vi "Main.vi"(10 "DAQ Type":enum16{"Hardware", "Simulation"}(ring), 11 "Module Admin":refnum<class "Delacor_lib_QMH_Module Admin.lvclass">) -> ()   [LabVIEW 2021, in "Serial Hardware.lvlib"]
doc: "This template is based off of the Queued Message Handler design pattern and the Queued Message Handler project template that ships with LabVIEW.\n\nThe main difference is that the queue is private to this module and communication between modules is performed via Broadcast and Request events.\n\nRequest events are wrapped in public API methods and are handled in the Event Handling Loop (EHL) of this VI. Any module can register for Broadcast events sent by this module. The EHL generates messages based on user interface actions.\n\nThe Message Handling Loop (MHL) processes messages generated by the EHL, or by other messages. The messages are string values, so new messages can be added easily to the Message Cases case structure in the MHL. Each message cluster can also provide an optional value for Message Data, which is a variant that can be converted to whatever message-specific data is required.\n_____\nBased on DQMH Project Template 6.1.0.94."
uses:
  Serial Hardware.lvlib
  <vilib>/Delacor/Delacor QMH/Libraries/Module Admin_class/Delacor_lib_QMH_Module Admin.lvclass
  Class/Serial Device/Serial Device.lvclass
  C:/repository/common_ATE/Libraries/Serial Hardware/Class/Abstract/Abstract.lvclass
  Message Data.ctl
  Class/Abstract/Abstract.lvclass
  Module Data--cluster.ctl
  Serial Parameter.ctl
  Write Data Command.ctl
  <vilib>/Delacor/Delacor QMH/Libraries/Message Queue_class/Delacor_lib_QMH_Message Queue.lvclass/Delacor_lib_QMH_Message Queue.ctl
  Stop Argument--cluster.ctl
  <vilib>/Delacor/Delacor QMH/Libraries/Module Admin_class/Delacor_lib_QMH_Module Admin.lvclass/Delacor_lib_QMH_Module Admin.ctl
  REQ Initialize Hardware Argument--cluster.ctl
  REQ Initialize Hardware (Reply Payload)--cluster.ctl
  REQ Acquire Data Argument--cluster.ctl
  REQ Close Ref Argument--cluster.ctl
  REQ Retry Argument--cluster.ctl
  REQ Write Command Argument--cluster.ctl
  REQ Start Logging Argument--cluster.ctl
  <vilib>/Utility/miscctls.llb/LVPointTypeDef.ctl
  User Interface/Instrument Address Command.ctl
  <vilib>/Delacor/Delacor QMH/Libraries/Message Queue_class/Delacor_lib_QMH_Enqueue Message (Single).vi
  <vilib>/Delacor/Delacor QMH/Libraries/Module Admin_class/Delacor_lib_QMH_Get External Launch.vi
  <vilib>/Utility/error.llb/Error Cluster From Error Code.vi
  <vilib>/ErrorRing/Error Ring.xnode
  <vilib>/Delacor/Delacor QMH/Libraries/Message Queue_class/Delacor_lib_QMH_Message Queue.lvclass
  User Interface/User Interface.lvlib
panel:
  out "error out":errorcluster
  out "Status":string
  in  "Simulate MHL Error":bool
  in  "Simulate EHL Error":bool
  # "Other QMH Modules communicate with this Module via its Public API (wrappers for its Request Events).\n\nThis Module communicates with other Modules via its Broadcast Events.\nAny module that wants to get these messages, just registers for this module's Broadcast events."
  # "This template is for the Delacor Modified Queued Message Handler design pattern.\n\nSee the block diagram for more information on how to use this template."
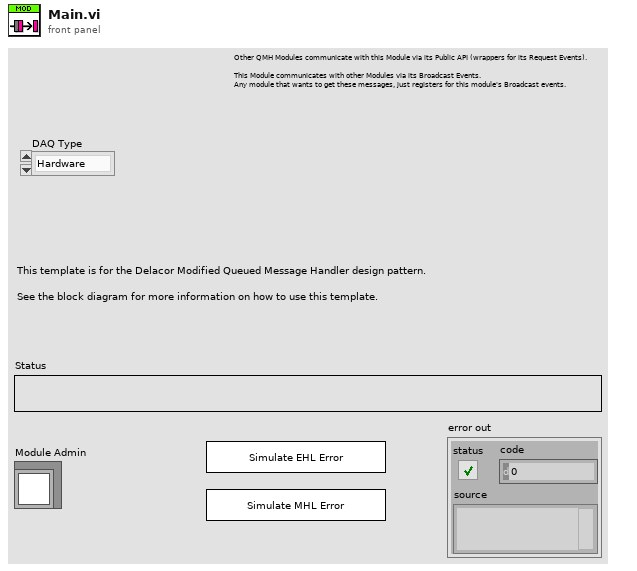
[diagram p1: front panel]
types:
  T1 = typedef "Serial Hardware.lvlib/Message Data.ctl" = cluster{"Message":string, "Data":string[]}
  T2 = typedef "Serial Hardware.lvlib/Request Events--cluster.ctl" = cluster{"Stop Module":refnum<user-event>, "Show Panel":refnum<user-event>, "Hide Panel":refnum<user-event>, "Get Module Execution Status":refnum<user-event>, "Show Diagram":refnum<user-event>, "REQ Initialize Hardware":refnum<user-event>, "REQ Wakeup_Helper_Loop":refnum<user-event>, "REQ Acquire Data":refnum<user-event>, "REQ Close Ref":refnum<user-event>, "REQ Retry":refnum<user-event>, "REQ Write Command":refnum<user-event>, "REQ Start Logging Helper Loop":refnum<user-event>, "REQ Start Logging":refnum<user-event>}
  T3 = typedef "Serial Hardware.lvlib/Write Data Command.ctl" = enum16{"Init", "Read", "Write", "close"}
  T4 = enum32{"invalid lock state", "Not Locked", "Locked (No Password)", "Password-protected"}
  T5 = typedef "Serial Hardware.lvlib/Stop Argument--cluster.ctl" = cluster{"Origin":string, "Exit via Stop Module Req?":bool, "Wait for Module to stop?":bool}
  T6 = typedef "Serial Hardware.lvlib/REQ Initialize Hardware Argument--cluster.ctl" = cluster{"Wait Notifier":refnum<notifier>, "wait for reply":bool}
  T7 = typedef "Serial Hardware.lvlib/REQ Acquire Data Argument--cluster.ctl" = cluster{"Boolean":bool}
  T8 = typedef "Serial Hardware.lvlib/REQ Close Ref Argument--cluster.ctl" = cluster{"Boolean":bool}
  T9 = typedef "Serial Hardware.lvlib/REQ Retry Argument--cluster.ctl" = cluster{"Boolean":bool}
  T10 = typedef "Serial Hardware.lvlib/REQ Write Command Argument--cluster.ctl" = cluster{"Command?":string}
  T11 = typedef "Serial Hardware.lvlib/REQ Start Logging Argument--cluster.ctl" = cluster{"Start Logging?":bool}
  T12 = typedef "User Interface.lvlib/Instrument Address Command.ctl" = enum16{"Init", "Read", "Write", "Close"}
  T13 = typedef "LVPointTypeDef.ctl" = cluster{"Horizontal":i16, "Vertical":i16}
  T14 = enum32{"Invalid", "Standard", "Closed", "Hidden", "Minimized", "Maximized"}
  T15 = typedef "Serial Hardware.lvlib/REQ Initialize Hardware (Reply Payload)--cluster.ctl" = cluster{"Connect?":bool, "error":errorcluster}
  T16 = typedef "Serial Hardware.lvlib/Module Data--cluster.ctl" = cluster{"Status":string, "File Path":path, "Serial Parameter":T17, "Abstract.lvclass":refnum<class "Abstract.lvclass">, "Start Logging?":bool}
  T17 = typedef "Serial Hardware.lvlib/Serial Parameter.ctl" = cluster{"VISA resource name":refnum<visa-resource-name>, "baud rate (9600)":u32, "data bits (8)":u16, "parity (0:none)":enum16{"None", "Odd", "Even", "Mark", "Space"}, "stop bits (10: 1 bit)":u16, "flow control (0:none)":u16, "termination char\n(0xA = '\\n' = LF) ":u8, "Enable Termination\nChar (T)":bool, "timeout (10sec)":u32}
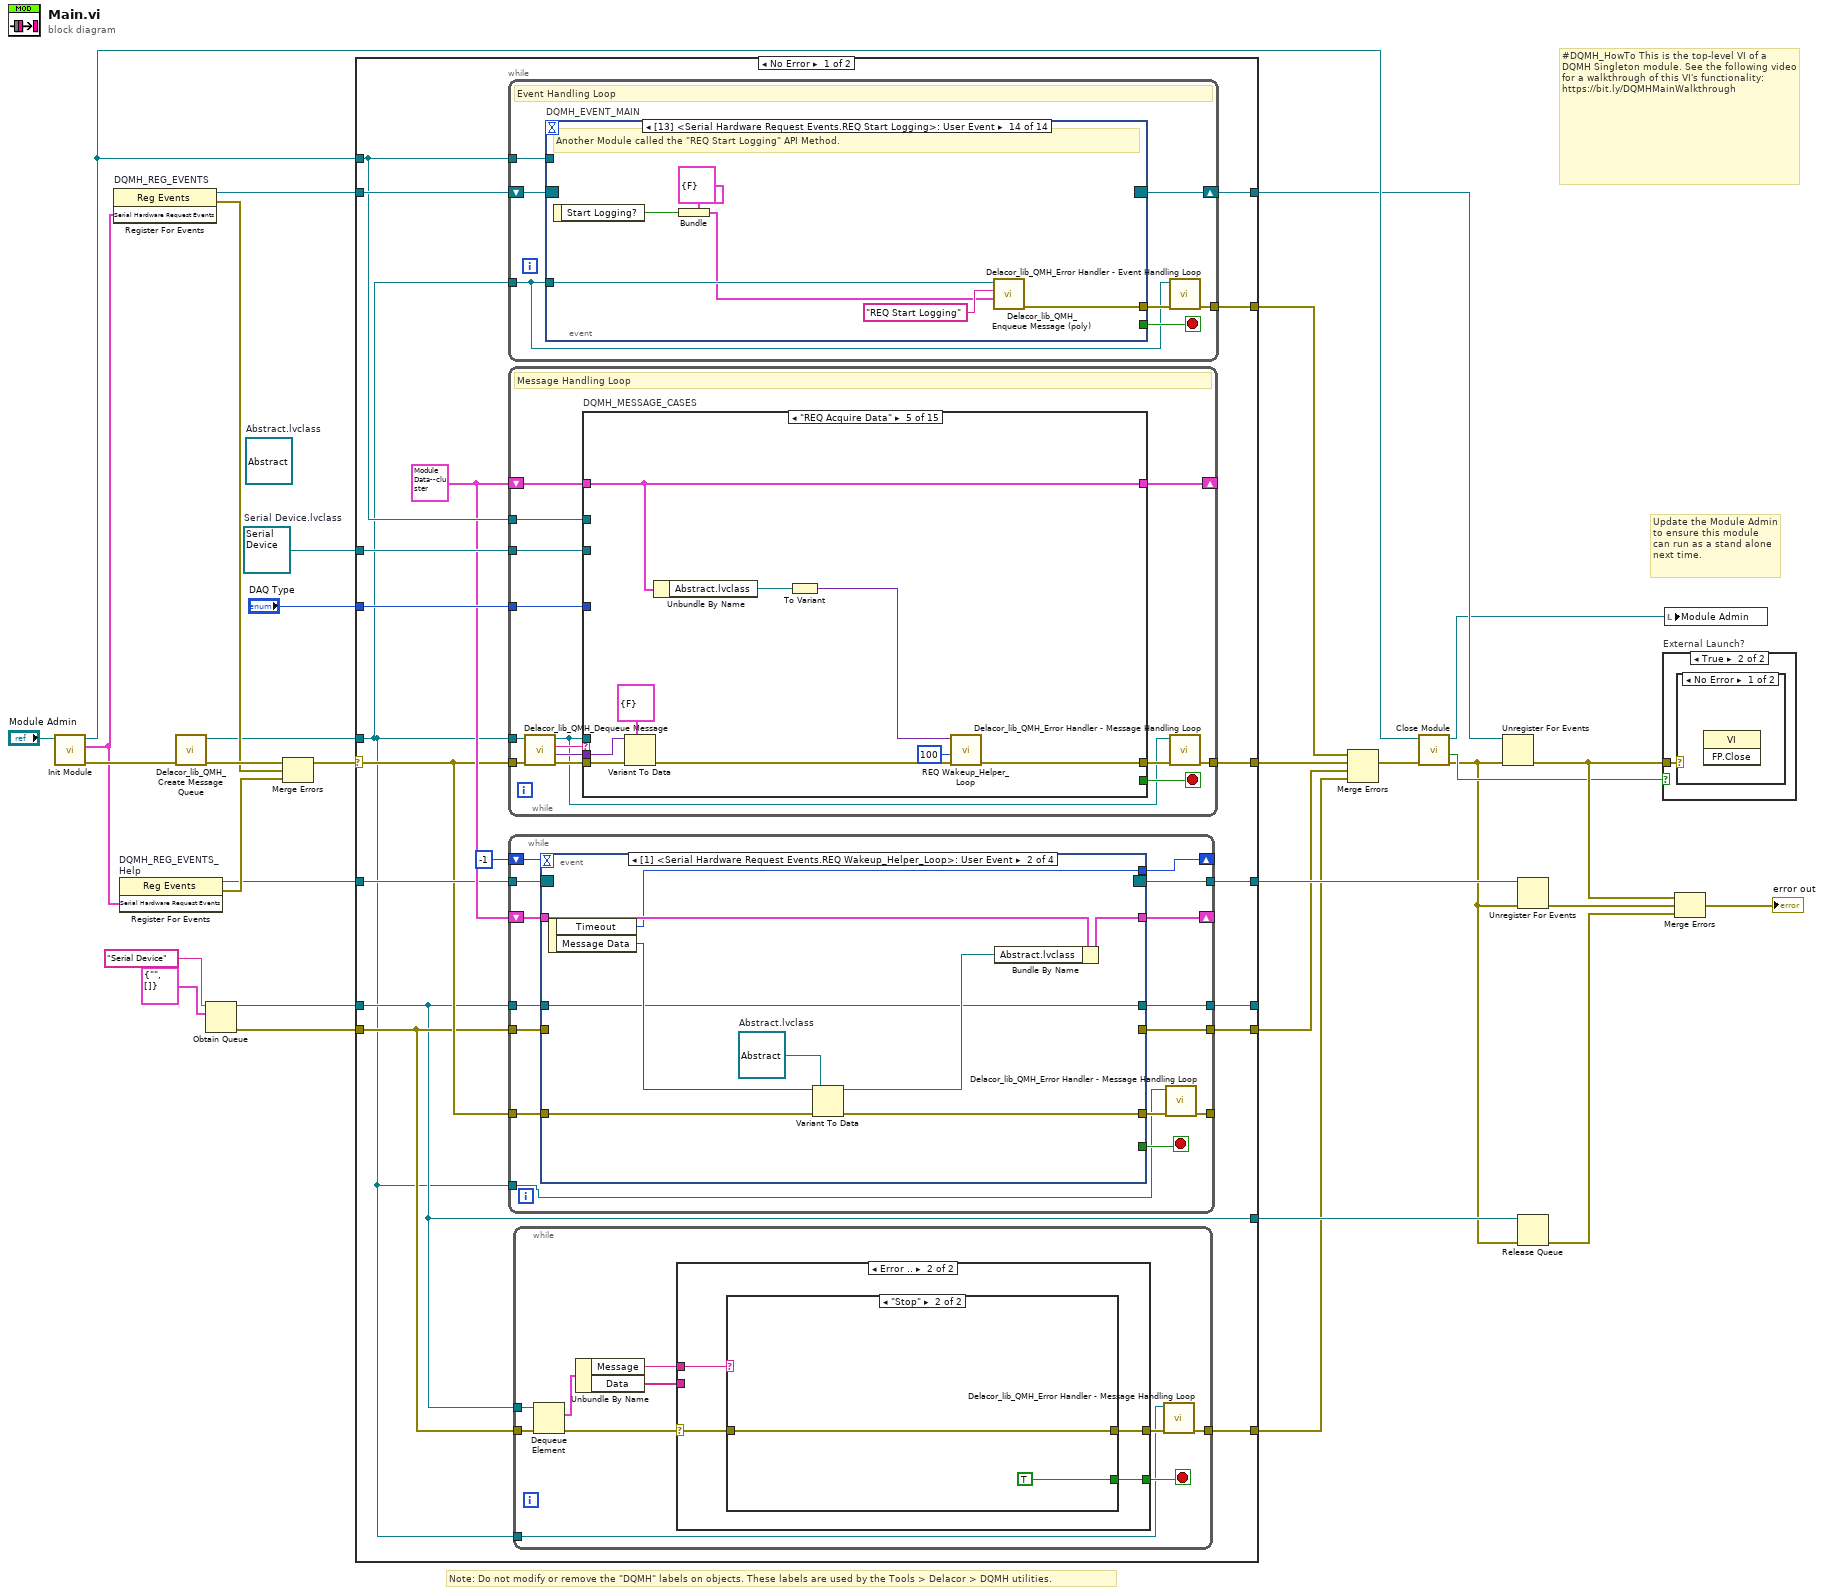
[diagram p0: block diagram]
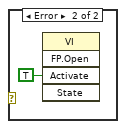
[diagram p3: hidden frame]
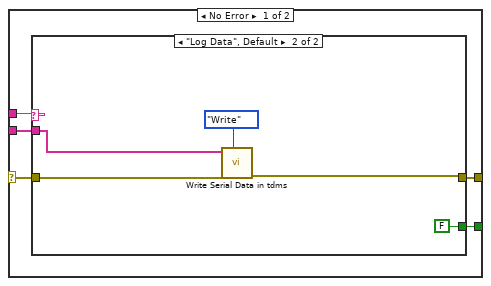
[diagram p4: hidden frame]
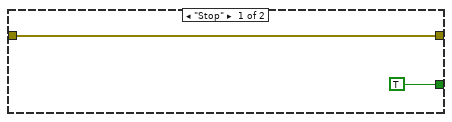
[diagram p5: hidden frame]
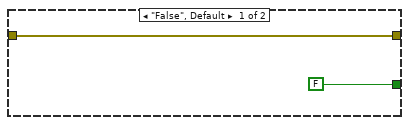
[diagram p6: hidden frame]
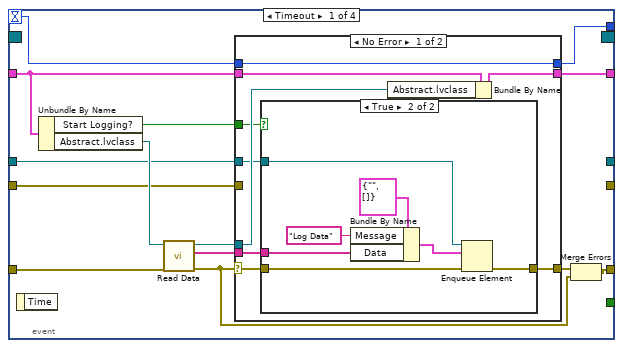
[diagram p7: hidden frame]
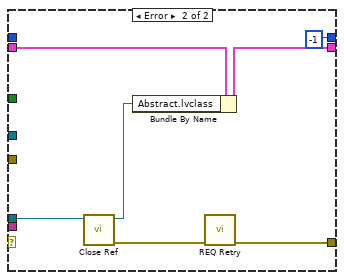
[diagram p9: hidden frame]
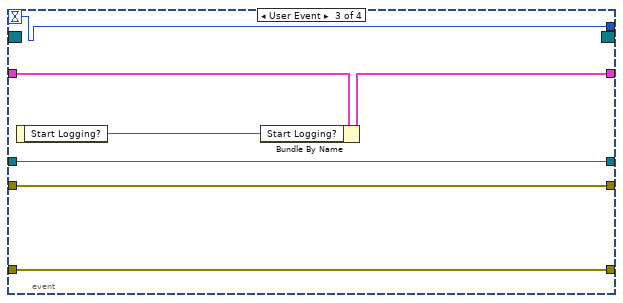
[diagram p10: hidden frame]
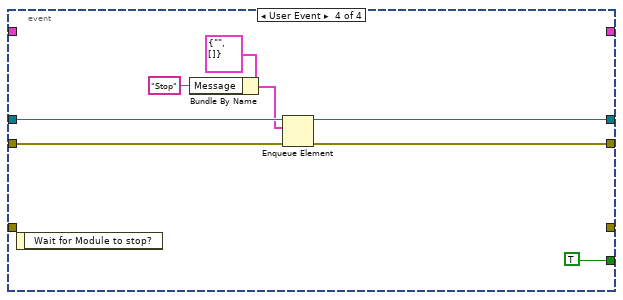
[diagram p11: hidden frame]
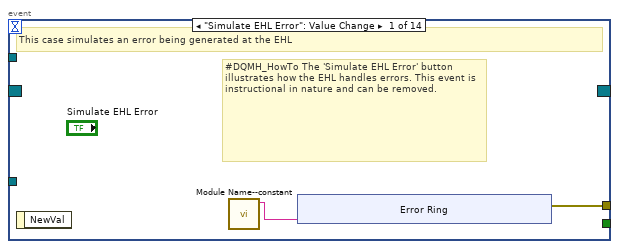
[diagram p12: hidden frame]
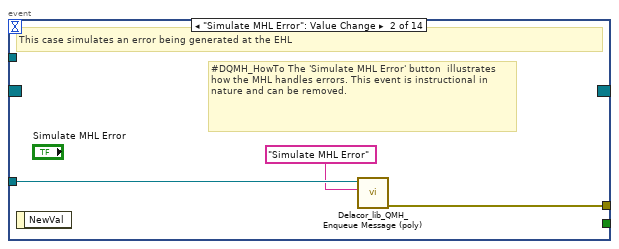
[diagram p13: hidden frame]
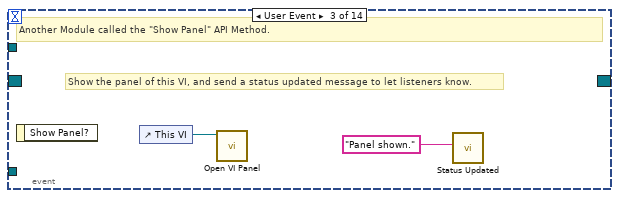
[diagram p14: hidden frame]
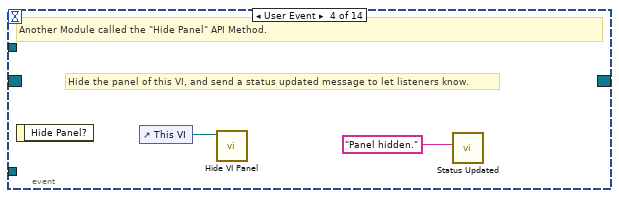
[diagram p15: hidden frame]
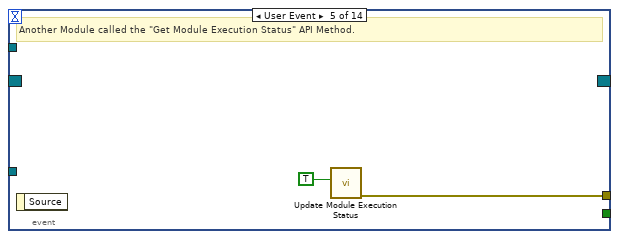
[diagram p16: hidden frame]
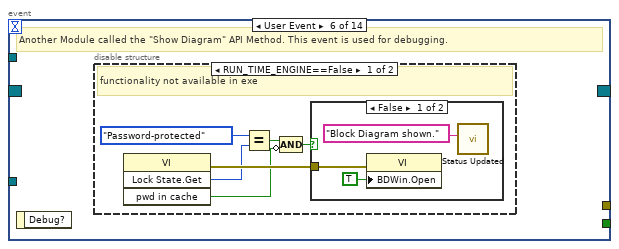
[diagram p17: hidden frame]
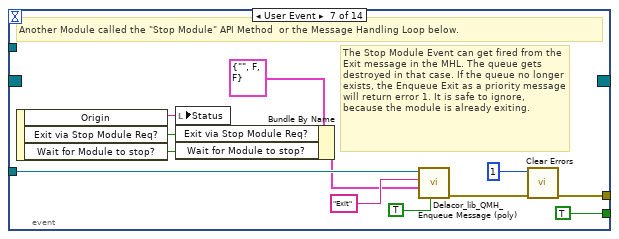
[diagram p20: hidden frame]
diagram:
  w17 = refnum<class "Serial Device.lvclass"> refnum  # Serial Device.lvclass
  (unwired) refnum<class "Abstract.lvclass"> refnum  # Abstract.lvclass
  # "#DQMH_HowTo This is the top-level VI of a DQMH Singleton module. See the following video for a walkthrough of this VI's functionality: https://bit.ly/DQMHMainWalkthrough"
  # "Note: Do not modify or remove the \"DQMH\" labels on objects. These labels are used by the Tools > Delacor > DQMH utilities."
  # "Update the Module Admin to ensure this module can run as a stand alone next time."
  n1 = call "Init Module.vi"("Singleton Module Admin in"="Module Admin") -> ("error out"=w31:errorcluster, "Serial Hardware Request Events"=w14:T2, "Singleton Module Admin out"=w24:refnum<class "Delacor_lib_QMH_Module Admin.lvclass">)  [unwired: 8 in]
  n2 = register-events "DQMH_REG_EVENTS"(w14) -> (reference out=w22:refnum<event-registration>, error out=w25:errorcluster)  [unwired: 2 in]
  n3 = register-events "DQMH_REG_EVENTS_Help"(w14) -> (reference out=w13:refnum<event-registration>, error out=w15:errorcluster)  [unwired: 2 in]
  n4 = call <vilib>:"Delacor_lib_QMH_Create Message Queue.vi"("error in"=w31) -> ("error out"=w27:errorcluster, "Message Queue"=w21:refnum<class "Delacor_lib_QMH_Message Queue.lvclass">)  [unwired: 9 in]
  n5 = Obtain Queue(name (unnamed)="Serial Device", element data type=T1 {"Message"="", "Data"=[]}) -> (queue out=w10:refnum<queue>, error out=w9:errorcluster)  [unwired: 3 in, 1 out]
  n6 = Merge Errors(w27, w25, w15) -> (w26:errorcluster)
  n7 = case shown="No Error" w26 {
    selector: w26 -> [w40 w454]
    tunnel: [w50 w453] -> w32
    tunnel: [w48 w459] -> w23
    tunnel: w22 -> [w47 w459]
    tunnel: w21 -> [w33 w452]
    tunnel: [w49 _] -> w30
    tunnel: w24 -> [w46 w455]
    tunnel: w17 -> [w45 _]
    tunnel: "DAQ Type" -> [w44 _]
    tunnel: w13 -> [w41 _]
    tunnel: w10 -> [w34 _]
    tunnel: w9 -> [w37 _]
    tunnel: [w39 _] -> _
    tunnel: [w38 _] -> w5
    tunnel: [w36 _] -> w8
    tunnel: [w35 _] -> w4
    tunnel: [w34 _] -> w7
    frame No Error {
      w43 = T16 {"Status"="", "File Path"=path "", "Serial Parameter"={"VISA resource name"="", "baud rate (9600)"=9600, "data bits (8)"=8, "parity (0:none)"=enum."None", "stop bits (10: 1 bit)"=10, "flow control (0:none)"=0, "termination char\n(0xA = '\\n' = LF) "=10, "Enable Termination\nChar (T)"=TRUE, "timeout (10sec)"=10000}, "Abstract.lvclass"=refnum, "Start Logging?"=FALSE} ("Data Cluster")
      n8 = while {
        tunnel: w33 -> [w158]
        shift-right: [w161] -> w48
        shift-left: w47 -> [w162]
        tunnel: [w163] -> w49
        tunnel: w46 -> [w159]
        stop <- w160 stop-if-true
        # "Event Handling Loop"
        n9 = event "DQMH_EVENT_MAIN" shown="[13] <Serial Hardware Request Events.REQ Start Logging>: User Event" {
          selector: w162 -> [_ _ _ _ _ _ _ _ _ _ _ _ _ _]
          dyn-events: [_ _ _ _ _ _ _ _ _ _ _ _ _ _] -> w161
          timeout: _ -> [_ _ _ _ _ _ _ _ _ _ _ _ _ _]
          tunnel: [_ _ _ _ _ _ TRUE ("Discard?") _ _ _ _ _ _ _] -> w160
          tunnel: w158 -> [_ w175 _ _ _ _ w199 w206 w220 w226 w232 w238 w244 w250]
          tunnel: [w166 w176 _ _ w182 _ w202 w208 w214 w221 w227 w233 w239 w245] -> w164
          tunnel: w159 -> [_ _ _ _ _ _ _ w205 _ _ _ _ _ _]
          event "Simulate EHL Error": Value Change {
            # "#DQMH_HowTo The 'Simulate EHL Error' button  illustrates how the EHL handles errors. This event is instructional in nature and can be removed."
            # "This case simulates an error being generated at the EHL"
            n10 = event-data() -> ()  [unwired: 1 in, 1 out]
            n11 = call "Module Name--constant.vi"() -> ("Module Name"=w165:string)  [unwired: 11 in]
            n12 = xnode "Error Ring"("parameter 0"=w165) -> ("error out"=w166:errorcluster)
          }
          event "Simulate MHL Error": Value Change {
            # "#DQMH_HowTo The 'Simulate MHL Error' button  illustrates how the MHL handles errors. This event is instructional in nature and can be removed."
            # "This case simulates an error being generated at the EHL"
            n13 = event-data() -> ()  [unwired: 1 in, 1 out]
            n14 = call-poly <vilib>:"Delacor_lib_QMH_Enqueue Message (poly).vi"("Message"="Simulate MHL Error", "Message Queue in"=w175) -> ("error out"=w176:errorcluster)  [unwired: 8 in, 1 out]
          }
          event User Event {
            # "Show the panel of this VI, and send a status updated message to let listeners know."
            # "Another Module called the \"Show Panel\" API Method."
            n15 = event-data() -> ()  [unwired: 1 in, 1 out]
            n16 = control-ref of="This VI"() -> (w178:refnum<vi>)
            n17 = call "Open VI Panel.vi"("VI"=w178) -> ()  [unwired: 10 in, 1 out]
            n18 = call "Status Updated.vi"("Status"="Panel shown." ("format string")) -> ()  [unwired: 10 in, 1 out]
          }
          event User Event {
            # "Hide the panel of this VI, and send a status updated message to let listeners know."
            # "Another Module called the \"Hide Panel\" API Method."
            n19 = event-data() -> ()  [unwired: 1 in, 1 out]
            n20 = control-ref of="This VI"() -> (w180:refnum<vi>)
            n21 = call "Hide VI Panel.vi"("VI"=w180) -> ()  [unwired: 10 in, 1 out]
            n22 = call "Status Updated.vi"("Status"="Panel hidden." ("format string")) -> ()  [unwired: 10 in, 1 out]
          }
          event User Event {
            # "Another Module called the \"Get Module Execution Status\" API Method."
            n23 = event-data() -> ()  [unwired: 1 in, 1 out]
            n24 = call "Update Module Execution Status.vi"("Running?"=TRUE) -> ("error out"=w182:errorcluster)  [unwired: 10 in]
          }
          event User Event {
            # "Another Module called the \"Show Diagram\" API Method. This event is used for debugging."
            n25 = event-data() -> ()  [unwired: 1 in, 1 out]
            n26 = disable-structure shown="RUN_TIME_ENGINE==False" {
              frame condition #0 (active) {
                # "functionality not available in exe"
                n27 = invoke class="VI" method="Lock State.Get"() -> (error out=w188:errorcluster, "Get Lock State"=w187:T4, "pwd in cache"=w184:bool)  [unwired: 4 in, 1 out]
                n28 = Equal?(x=T4."Password-protected", y=w187) -> (x = y?=w185:bool)
                n29 = Compound Arithmetic op=AND(w185, invert w184) -> (w183:bool)
                n30 = case shown="False" w183 {
                  tunnel: w188 -> [w191 _]
                  frame False {
                    n31 = property class="VI"(error in=w191, "BDWin.Open"=TRUE ("Block Diagram Window:Open")) -> ()  [unwired: 1 in, 2 out]
                    n32 = call "Status Updated.vi"("Status"="Block Diagram shown." ("format string")) -> ()  [unwired: 10 in, 1 out]
                  }
                  frame True {
                    # "Password-protected VI, and the password is not in the cache. Do not show the diagram."
                  }
                }
              }
              frame condition #1 {
              }
            }
          }
          event User Event {
            # "The Stop Module Event can get fired from the Exit message in the MHL. The queue gets destroyed in that case. If the queue no longer exists, the Enqueue Exit as a priority message will return error 1. It is safe to ignore, because the module is already exiting."
            # "Another Module called the \"Stop Module\" API Method  or the Message Handling Loop below."
            n33 = event-data() -> ("Origin"=w198:string, "Exit via Stop Module Req?"=w194:bool, "Wait for Module to stop?"=w193:bool)  [unwired: 1 in]
            n34 = local write "Status"(w198) -> ()
            n35 = Bundle By Name(cluster=T5 {"Origin"="", "Exit via Stop Module Req?"=FALSE, "Wait for Module to stop?"=FALSE} ("Stop Argument"), "Exit via Stop Module Req?"=w194, "Wait for Module to stop?"=w193) -> (w192:T5)
            n36 = call-poly <vilib>:"Delacor_lib_QMH_Enqueue Message (poly).vi"("Priority Message? (F)"=TRUE, "Message Data"=w192, "Message"="Exit", "Message Queue in"=w199) -> ("error out"=w203:errorcluster)  [unwired: 6 in, 1 out]
            n37 = call <vilib>:"Clear Errors.vi"("error in (no error)"=w203, "specific error code to clear (0: all)"=1) -> ("error out"=w202:errorcluster)  [unwired: 4 in, 1 out]
          }
          event Panel Close? {
            w207 = TRUE  # Discard the event, the MHL is responsible for closing and stopping this VI.
            # "Hide the panel or send the 'Exit' message if the user clicks the 'X' on the module main VI panel."
            n38 = event-data() -> ()  [unwired: 1 in, 1 out]
            n39 = property class="Module Admin"(reference=w205) -> ("Accessors:External Launch"=w204:bool)  [unwired: 1 in, 2 out]
            n40 = case shown="False" w204 {
              tunnel: w206 -> [_ w212]
              tunnel: [_ w213] -> w208
              frame True {
                # "If externally launched, clicking the 'X' hides the panel, but doesn't close it."
                n41 = control-ref of="This VI"() -> (w209:refnum<vi>)
                n42 = call "Hide VI Panel.vi"("VI"=w209) -> ()  [unwired: 10 in, 1 out]
              }
              frame False {
                # "If run as a stand-alone VI, clicking the panel 'X' stops the VI."
                n43 = call-poly <vilib>:"Delacor_lib_QMH_Enqueue Message (poly).vi"("Priority Message? (F)"=TRUE, "Message"="Exit", "Message Queue in"=w212) -> ("error out"=w213:errorcluster)  [unwired: 7 in, 1 out]
              }
            }
            n44 = event-data("Discard?"=w207) -> ()  [unwired: 1 in, 1 out]
          }
          event User Event {
            # "Another Module called the \"REQ Initialize Hardware\" API Method."
            n45 = event-data() -> ("Wait Notifier"=w216:refnum<notifier>, "wait for reply"=w215:bool)  [unwired: 1 in]
            n46 = Bundle(cluster=T6 {"Wait Notifier"=refnum, "wait for reply"=FALSE} ("REQ Initialize Hardware Argument"), "Wait Notifier"=w216, "wait for reply"=w215) -> (w217:T6)
            n47 = call-poly <vilib>:"Delacor_lib_QMH_Enqueue Message (poly).vi"("Message Data"=w217, "Message"="REQ Initialize Hardware", "Message Queue in"=w220) -> ("error out"=w214:errorcluster)  [unwired: 7 in, 1 out]
          }
          event User Event {
            # "Another Module called the \"REQ Acquire Data\" API Method."
            n48 = event-data() -> ("Boolean"=w222:bool)  [unwired: 1 in]
            n49 = Bundle(cluster=T7 {"Boolean"=FALSE} ("REQ Acquire Data Argument"), "Boolean"=w222) -> (w223:T7)
            n50 = call-poly <vilib>:"Delacor_lib_QMH_Enqueue Message (poly).vi"("Message Data"=w223, "Message"="REQ Acquire Data", "Message Queue in"=w226) -> ("error out"=w221:errorcluster)  [unwired: 7 in, 1 out]
          }
          event User Event {
            # "Another Module called the \"REQ Close Ref\" API Method."
            n51 = event-data() -> ("Boolean"=w228:bool)  [unwired: 1 in]
            n52 = Bundle(cluster=T8 {"Boolean"=FALSE} ("REQ Close Ref Argument"), "Boolean"=w228) -> (w229:T8)
            n53 = call-poly <vilib>:"Delacor_lib_QMH_Enqueue Message (poly).vi"("Message Data"=w229, "Message"="REQ Close Ref", "Message Queue in"=w232) -> ("error out"=w227:errorcluster)  [unwired: 7 in, 1 out]
          }
          event User Event {
            # "Another Module called the \"REQ Retry\" API Method."
            n54 = event-data() -> ("Boolean"=w234:bool)  [unwired: 1 in]
            n55 = Bundle(cluster=T9 {"Boolean"=FALSE} ("REQ Retry Argument"), "Boolean"=w234) -> (w235:T9)
            n56 = call-poly <vilib>:"Delacor_lib_QMH_Enqueue Message (poly).vi"("Message Data"=w235, "Message"="REQ Retry", "Message Queue in"=w238) -> ("error out"=w233:errorcluster)  [unwired: 7 in, 1 out]
          }
          event User Event {
            # "Another Module called the \"REQ Write Command\" API Method."
            n57 = event-data() -> ("Command?"=w240:string)  [unwired: 1 in]
            n58 = Bundle(cluster=T10 {"Command?"=""} ("REQ Write Command Argument"), "Command?"=w240) -> (w241:T10)
            n59 = call-poly <vilib>:"Delacor_lib_QMH_Enqueue Message (poly).vi"("Message Data"=w241, "Message"="REQ Write Command", "Message Queue in"=w244) -> ("error out"=w239:errorcluster)  [unwired: 7 in, 1 out]
          }
          event User Event {
            # "Another Module called the \"REQ Start Logging\" API Method."
            n60 = event-data() -> ("Start Logging?"=w246:bool)  [unwired: 1 in]
            n61 = Bundle(cluster=T11 {"Start Logging?"=FALSE} ("REQ Start Logging Argument"), "Start Logging?"=w246) -> (w247:T11)
            n62 = call-poly <vilib>:"Delacor_lib_QMH_Enqueue Message (poly).vi"("Message Data"=w247, "Message"="REQ Start Logging", "Message Queue in"=w250) -> ("error out"=w245:errorcluster)  [unwired: 7 in, 1 out]
          }
        }
        n63 = call-dynamic "Delacor_lib_QMH_Error Handler - Event Handling Loop.vi"("error in"=w164, "Message Queue in"=w158) -> ("dup error in"=w163:errorcluster)  [unwired: 8 in, 1 out]
      }
      n64 = while {
        tunnel: w33 -> [w255]
        shift-right: [w259] -> _
        shift-left: w43 -> [w260]
        tunnel: w40 -> [w263]
        tunnel: [w261] -> w50
        tunnel: w46 -> [w253]
        tunnel: w45 -> [w252]
        tunnel: w44 -> [w251]
        stop <- w258 stop-if-true
        # "Message Handling Loop"
        n65 = call-dynamic "Delacor_lib_QMH_Dequeue Message.vi"("error in"=w263, "Message Queue in"=w255) -> ("error out"=w262:errorcluster, "Message Data"=w256:variant, "Message"=w257:string, "Message Queue out"=w254:refnum<class "Delacor_lib_QMH_Message Queue.lvclass">)  [unwired: 6 in]
        n66 = case "DQMH_MESSAGE_CASES" shown="\"REQ Acquire Data\"" w257 {
          selector: w257 -> [_ _ _ _ _ _ _ _ _ _ _ _ _ _ w439]
          tunnel: w254 -> [w269 _ _ _ _ _ w347 _ _ _ _ _ w409 w431 _]
          tunnel: w262 -> [w290 w300 w303 w321 w332 w341 w357 w376 w385 w392 w394 w399 w416 w437 w441]
          tunnel: [w266 w295 w303 w308 w328 w337 w349 w366 w377 w391 w394 w398 w412 w434 w442] -> w264
          tunnel: w260 -> [w280 w299 w302 w312 w327 w336 w352 w370 w384 w390 w393 w396 w411 w430 w440]
          tunnel: [w279 w294 w302 w310 w327 w334 w344 w368 w384 w390 w393 w396 w411 w430 w440] -> w259
          tunnel: [_ _ _ _ _ _ _ _ _ _ _ _ _ w429 _] -> w258
          tunnel: w256 -> [_ _ _ w320 w331 w340 w356 w375 w383 _ _ _ w410 w428 _]
          tunnel: w253 -> [w281 _ _ _ _ _ _ _ _ _ _ _ w408 w423 _]
          tunnel: w252 -> [w265 _ _ _ _ _ _ _ _ _ _ _ _ _ _]
          tunnel: w251 -> [_ _ _ w304 _ _ w353 _ _ _ _ _ _ _ _]
          frame "Initialize" {
            w275 = "Initial Message" ("Initial Message")
            # "Initialize - Any operation that needs to be done before the module can receive messages. Synchronize Caller Events.vi will inform Start Module.vi that the module has launched and is ready to receive messages. Module Did Init.vi will broadcast that the module initialized."
            n67 = call "Synchronize Caller Events.vi"("error in (no error)"=w290, "Singleton Module Admin in"=w281) -> ("error out"=w289:errorcluster, "Singleton Module Admin out"=w276:refnum<class "Delacor_lib_QMH_Module Admin.lvclass">)  [unwired: 8 in]
            n68 = property on="Pane" class="Pane"("Origin"=T13 {"Horizontal"=0, "Vertical"=0}) -> ()  [unwired: 2 in, 2 out]
            n69 = property class="Module Admin"(reference=w276) -> ("Accessors:External Launch"=w285:bool)  [unwired: 1 in, 2 out]
            n70 = call "Module Name--constant.vi"() -> ("Module Name"=w288:string)  [unwired: 11 in]
            n71 = call "Module Name--constant.vi"() -> ("Module Name"=w277:string)  [unwired: 11 in]
            n72 = property class="VI"("Front Panel.Title"=w288) -> (reference out=w287:refnum<vi>, error out=w292:errorcluster)  [unwired: 2 in]
            n73 = Select(t=T14."Hidden" ("State"), s=w285, f=T14."Standard" ("State")) -> (s? t:f=w282:T14)
            n74 = call "Module Did Init.vi"("error in (no error)"=w289, "Initialized?"=TRUE, "Origin"=w277) -> ("error out"=w272:errorcluster)  [unwired: 8 in]
            n75 = invoke class="VI" method="FP.Open"(reference=w287, error in=w292, "State"=w282) -> (reference out=w286:refnum<vi>, error out=w291:errorcluster)  [unwired: 2 in, 3 out]
            n76 = invoke class="VI" method="FP.Center"(reference=w286, error in=w291) -> ()  [unwired: 1 in, 3 out]
            n77 = call "Instrument Address.vi"("Command"=Instrument_Address_Command."Init", "error in (no error)"=w272, "name or relative path"="Serial.ini") -> ("error out"=w267:errorcluster, "path_out"=w270:path)  [unwired: 6 in, 1 out]
            n78 = Bundle By Name(cluster=w280, "Status"=w275, "Abstract.lvclass"=w265, "File Path"=w270) -> (w279:T16)
            n79 = call-poly <vilib>:"Delacor_lib_QMH_Enqueue Message (poly).vi"("error in"=w267, "Message"="REQ Inst Address", "Message Queue in"=w269) -> ("error out"=w266:errorcluster)  [unwired: 7 in, 1 out]
            "Status" <- w275
          }
          frame "REQ Inst Address" {
            n80 = Unbundle By Name(w299) -> ("File Path"=w298:path)
            n81 = call "Instrument Address.vi"("Command"=Instrument_Address_Command."Read", "error in (no error)"=w300, "path_in"=w298) -> ("error out"=w297:errorcluster, "Instrument Parameter"=w296:string[][])  [unwired: 6 in, 1 out]
            n82 = call "Read Serial Setting.vi"("error in (no error)"=w297, "Device Parameter"=w296) -> ("error out"=w295:errorcluster, "Serial Parameetr"=w293:T17)  [unwired: 8 in]
            n83 = Bundle By Name(cluster=w299, "Serial Parameter"=w293) -> (w294:T16)
          }
          frame "---Module Specific---" {
            # "Separator -- The following cases handle messages specific to this Module."
          }
          frame "REQ Initialize Hardware" {
            n84 = Variant To Data(error in=w321, type=T6 {"Wait Notifier"=refnum, "wait for reply"=FALSE} ("REQ Initialize Hardware Argument"), Variant=w320) -> (data=w318:T6, error out=w313:errorcluster)
            n85 = Unbundle By Name(w318) -> ("Wait Notifier"=w317:refnum<notifier>, "wait for reply"=w316:bool)
            n86 = Unbundle By Name(w312) -> ("Abstract.lvclass"=w311:refnum<class "Abstract.lvclass">, "Serial Parameter"=w305:T17)
            n87 = call-dynamic "Initialize Hardware.vi"("error in (no error)"=w313, "DAQ Type"=w304, "Serial Parameter"=w305, "Abstract in"=w311) -> ("error out"=w308:errorcluster, "Abstract out"=w309:refnum<class "Abstract.lvclass">)  [unwired: 6 in]
            n88 = Unbundle By Name(w308) -> ("status"=w307:bool)
            n89 = Bundle By Name(cluster=w312, "Abstract.lvclass"=w309) -> (w310:T16)
            n90 = Not(x=w307) -> (.not. x?=w306:bool)
            n91 = Bundle By Name(cluster=T15 {"Connect?"=FALSE, "error"={"status"=FALSE, "code"=0, "source"=""}} ("REQ Initialize Hardware (Reply Payload)"), "Connect?"=w306) -> (w315:T15)
            n92 = case shown="True" w316 {
              tunnel: w317 -> [_ w323]
              tunnel: w315 -> [_ w322]
              frame False {
              }
              frame True {
                n93 = Send Notification(notification=w322, notifier=w323) -> ()  [unwired: 1 in, 2 out]
              }
            }
          }
          frame "REQ Acquire Data" {
            n94 = Variant To Data(error in=w332, type=T7 {"Boolean"=FALSE} ("REQ Acquire Data Argument"), Variant=w331) -> (error out=w329:errorcluster)  [unwired: 1 out]
            n95 = Unbundle By Name(w327) -> ("Abstract.lvclass"=w326:refnum<class "Abstract.lvclass">)
            n96 = To Variant(anything=w326) -> (Variant=w325:variant)
            n97 = call "REQ Wakeup_Helper_Loop.vi"("error in"=w329, "Timeout"=100, "Message Data"=w325) -> ("error out"=w328:errorcluster)  [unwired: 8 in]
          }
          frame "REQ Close Ref" {
            n98 = Variant To Data(error in=w341, type=T8 {"Boolean"=FALSE} ("REQ Close Ref Argument"), Variant=w340) -> (error out=w338:errorcluster)  [unwired: 1 out]
            n99 = Unbundle By Name(w336) -> ("Abstract.lvclass"=w335:refnum<class "Abstract.lvclass">)
            n100 = call-dynamic "Close Ref.vi"("error in (no error)"=w338, "Abstract in"=w335) -> ("error out"=w337:errorcluster, "Abstract out"=w333:refnum<class "Abstract.lvclass">)  [unwired: 8 in]
            n101 = Bundle By Name(cluster=w336, "Abstract.lvclass"=w333) -> (w334:T16)
          }
          frame "REQ Retry" {
            n102 = Unbundle By Name(w352) -> ("Abstract.lvclass"=w351:refnum<class "Abstract.lvclass">, "Serial Parameter"=w350:T17)
            n103 = Variant To Data(error in=w357, type=T9 {"Boolean"=FALSE} ("REQ Retry Argument"), Variant=w356) -> (error out=w354:errorcluster)  [unwired: 1 out]
            n104 = call-dynamic "Initialize Hardware.vi"("error in (no error)"=w354, "DAQ Type"=w353, "Serial Parameter"=w350, "Abstract in"=w351) -> ("error out"=w345:errorcluster, "Abstract out"=w348:refnum<class "Abstract.lvclass">)  [unwired: 6 in]
            n105 = Wait (ms)(milliseconds to wait=u32 2000) -> ()  [unwired: 1 out]
            n106 = case shown="No Error" w345 {
              selector: w345 -> [w359 _]
              tunnel: w348 -> [w358 w365]
              tunnel: w347 -> [_ w362]
              tunnel: [w359 w361] -> w346
              tunnel: [w358 w360] -> w343
              frame No Error {
              }
              frame Error {
                n107 = call-dynamic "Close Ref.vi"("Abstract in"=w365) -> ("error out"=w363:errorcluster, "Abstract out"=w360:refnum<class "Abstract.lvclass">)  [unwired: 9 in]
                n108 = call-poly <vilib>:"Delacor_lib_QMH_Enqueue Message (poly).vi"("error in"=w363, "Message"="REQ Retry", "Message Queue in"=w362) -> ("error out"=w361:errorcluster)  [unwired: 7 in, 1 out]
              }
            }
            n109 = Bundle By Name(cluster=w352, "Abstract.lvclass"=w343) -> (w344:T16)
            n110 = Merge Errors(w345, w346) -> (w349:errorcluster)
          }
          frame "REQ Write Command" {
            n111 = Variant To Data(error in=w376, type=T10 {"Command?"=""} ("REQ Write Command Argument"), Variant=w375) -> (data=w373:T10, error out=w372:errorcluster)
            n112 = Unbundle By Name(w373) -> ("Command?"=w371:string)
            n113 = Unbundle By Name(w370) -> ("Abstract.lvclass"=w369:refnum<class "Abstract.lvclass">)
            n114 = call-dynamic "Write Command.vi"("error in (no error)"=w372, "Command?"=w371, "Abstract in"=w369) -> ("error out"=w366:errorcluster, "Abstract out"=w367:refnum<class "Abstract.lvclass">)  [unwired: 7 in]
            n115 = Bundle By Name(cluster=w370, "Abstract.lvclass"=w367) -> (w368:T16)
          }
          frame "REQ Start Logging" {
            n116 = Variant To Data(error in=w385, type=T11 {"Start Logging?"=FALSE} ("REQ Start Logging Argument"), Variant=w383) -> (data=w381:T11, error out=w380:errorcluster)
            n117 = Unbundle By Name(w381) -> ("Start Logging?"=w378:bool)
            n118 = call "REQ Start Logging Helper Loop.vi"("error in"=w380, "Start Logging?"=w378) -> ("error out"=w379:errorcluster)  [unwired: 9 in]
            n119 = case shown="True" w378 {
              tunnel: w379 -> [w386 w388]
              tunnel: [w386 w387] -> w377
              frame False {
              }
              frame True {
                n120 = call "Write Serial Data in tdms.vi"("Command"=Write_Data_Command."Init", "error in (no error)"=w388) -> ("error out"=w387:errorcluster)  [unwired: 9 in]
              }
            }
          }
          frame "---Copy This Frame---" {
            # "Duplicate this frame when creating new messages.  Change this comment in the duplicated frame to describe this message."
            n121 = Merge Errors(w392) -> (w391:errorcluster)
          }
          frame "---Exit and Error Handling---" {
            # "Separator - The following cases handle errors and exit messages."
          }
          frame "Simulate MHL Error" {
            # "#DQMH_HowTo The 'Simulate MHL Error' button  illustrates how the MHL handles errors. This event is instructional in nature and can be removed."
            # "Simulate an error occurring at the MHL"
            n122 = call "Module Name--constant.vi"() -> ("Module Name"=w395:string)  [unwired: 11 in]
            n123 = xnode "Error Ring"("parameter 0"=w395) -> ("error out"=w397:errorcluster)
            n124 = Merge Errors(w399, w397) -> (w398:errorcluster)
          }
          frame "Error" {
            # "#CodeRecommended - If you ever change the name of this \"Error\" message, you'll need to update the name in the Check Loop Error.vi as well."
            # "#CodeRecommended - If the module is running in standalone mode (External Launch = FALSE), this code will pop up an error dialog and call the 'Exit' message if an error occurs. Add more fine-grained error handling here."
            # "Error - Check the error message data and respond accordingly. This message is sent by the \"Error Handler\" VIs at the end of each loop in this application."
            n125 = property class="Module Admin"(reference=w408) -> ("Accessors:External Launch"=w407:bool)  [unwired: 1 in, 2 out]
            n126 = Variant To Data(error in=w416, type=errorcluster {"status"=FALSE, "code"=0, "source"=""} ("error constant"), Variant=w410) -> (data=w417:errorcluster, error out=w414:errorcluster)
            n127 = call "Error Reported.vi"("Error"=w417) -> ()  [unwired: 10 in, 1 out]
            n128 = case shown="False" w407 {
              tunnel: [w422 _] -> w413
              tunnel: w409 -> [w420 _]
              tunnel: w417 -> [w421 _]
              frame False {
                # "If the module is running standalone, then pop up an error dialog and call the \"Exit\" message."
                n129 = call <vilib>:"Simple Error Handler.vi"("error in (no error)"=w421) -> ()  [unwired: 4 in, 5 out]
                n130 = call-poly <vilib>:"Delacor_lib_QMH_Enqueue Message (poly).vi"("Priority Message? (F)"=TRUE, "Message"="Exit", "Message Queue in"=w420) -> ("error out"=w422:errorcluster)  [unwired: 7 in, 1 out]
              }
              frame True {
                # "If the module was launched externally, calling the Error Reported broadcast VI is the only action performed by the \"Error\" message. The module's caller can then process the error appropriately."
              }
            }
            n131 = Merge Errors(w414, w413) -> (w412:errorcluster)
            n132 = local write "error out"(w412) -> ()
          }
          frame "Exit" {
            w427 = 91  # 91: not all Exit messages will have an argument
            w429 = TRUE  # Stop the VI
            # "Release the message queue reference"
            # "#CodeNeeded - Add any required cleanup code here"
            # "Exit - Exit the application."
            n133 = Variant To Data(error in=w437, type=T5 {"Origin"="", "Exit via Stop Module Req?"=FALSE, "Wait for Module to stop?"=FALSE} ("Stop Argument"), Variant=w428) -> (data=w425:T5, error out=w433:errorcluster)
            n134 = call <vilib>:"Clear Errors.vi"("error in (no error)"=w433, "specific error code to clear (0: all)"=w427) -> ("error out"=w436:errorcluster)  [unwired: 4 in, 1 out]
            n135 = control-ref of="This VI"() -> (w424:refnum<vi>)
            n136 = call-dynamic "Delacor_lib_QMH_Release Message Queue.vi"("error in"=w436, "Message Queue"=w431) -> ("error out"=w435:errorcluster)  [unwired: 9 in]
            n137 = call "Handle Exit.vi"("Stop Argument"=w425, "Admin in"=w423, "VI reference"=w424) -> ("error out"=w432:errorcluster)  [unwired: 7 in, 1 out]
            n138 = Merge Errors(w435, w432) -> (w434:errorcluster)
          }
          frame Default {
            # "'Default' case only runs if there is a message that isn't defined in any of the other cases.  Output a programming error."
            n139 = call "Module Name--constant.vi"() -> ("Module Name"=w438:string)  [unwired: 11 in]
            n140 = xnode "Error Ring"("parameter 0"=w439, "parameter 1"=w438) -> ("error out"=w443:errorcluster)
            n141 = Merge Errors(w441, w443) -> (w442:errorcluster)
          }
        }
        n142 = call-dynamic "Delacor_lib_QMH_Error Handler - Message Handling Loop.vi"("error in"=w264, "Message Queue in"=w254) -> ("dup error in"=w261:errorcluster)  [unwired: 8 in, 1 out]
      }
      n143 = while {
        shift-right: [w90] -> _
        shift-left: w43 -> [w95]
        shift-right: [w89] -> _
        shift-left: -1 -> [w94]
        tunnel: w41 -> [w93]
        tunnel: w40 -> [w92]
        tunnel: [w87] -> _
        tunnel: w33 -> [w86]
        tunnel: w34 -> [w85]
        tunnel: w37 -> [w84]
        tunnel: [w83] -> w39
        tunnel: [w82] -> w38
        tunnel: [w81] -> w36
        stop <- w91 stop-if-true
        n144 = event shown="[1] <Serial Hardware Request Events.REQ Wakeup_Helper_Loop>: User Event" {
          selector: w93 -> [_ _ _ _]
          dyn-events: [_ _ _ _] -> w81
          timeout: w94 -> [w108 _ w143 _]
          tunnel: w95 -> [w105 w139 w149 _]
          tunnel: w92 -> [w109 w142 w148 _]
          tunnel: [_ _ _ TRUE] -> w91
          tunnel: [w106 w138 w147 _] -> w90
          tunnel: [w102 w136 w148 _] -> w88
          tunnel: [w107 w135 w143 _] -> w89
          tunnel: w85 -> [w99 w134 w145 w156]
          tunnel: w84 -> [w98 _ w144 w155]
          tunnel: [_ w134 w145 w151] -> w83
          tunnel: [_ _ w144 w150] -> w82
          event Timeout {
            n145 = event-data() -> ()  [unwired: 1 in, 1 out]
            n146 = Unbundle By Name(w105) -> ("Start Logging?"=w97:bool, "Abstract.lvclass"=w104:refnum<class "Abstract.lvclass">)
            n147 = call-dynamic "Read Data.vi"("error in (no error)"=w109, "Abstract in"=w104) -> ("error out"=w100:errorcluster, "Channel Data"=w96:string[], "Abstract out"=w103:refnum<class "Abstract.lvclass">)  [unwired: 7 in]
            n148 = case shown="No Error" w100 {
              selector: w100 -> [w112 _]
              tunnel: w108 -> [w118 _]
              tunnel: [w118 -1] -> w107
              tunnel: [w116 w130] -> w106
              tunnel: w105 -> [w117 w132]
              tunnel: w103 -> [w115 w131]
              tunnel: [w111 w127] -> w101
              tunnel: w99 -> [w114 _]
              tunnel: w98 -> [_ _]
              tunnel: w97 -> [w113 _]
              tunnel: w96 -> [w110 _]
              frame No Error {
                n149 = case shown="True" w113 {
                  tunnel: w114 -> [_ w126]
                  tunnel: w112 -> [w119 w125]
                  tunnel: [w119 w124] -> w111
                  tunnel: w110 -> [_ w120]
                  frame False {
                  }
                  frame True {
                    n150 = Bundle By Name(cluster=T1 {"Message"="", "Data"=[]}, "Message"="Log Data", "Data"=w120) -> (w122:T1)
                    n151 = Enqueue Element(queue=w126, element=w122, error in (no error)=w125) -> (error out=w124:errorcluster)  [unwired: 1 in, 2 out]
                  }
                }
                n152 = Bundle By Name(cluster=w117, "Abstract.lvclass"=w115) -> (w116:T16)
              }
              frame Error {
                n153 = call-dynamic "Close Ref.vi"("Abstract in"=w131) -> ("error out"=w128:errorcluster, "Abstract out"=w129:refnum<class "Abstract.lvclass">)  [unwired: 9 in]
                n154 = Bundle By Name(cluster=w132, "Abstract.lvclass"=w129) -> (w130:T16)
                n155 = call "REQ Retry.vi"("error in"=w128) -> ("error out"=w127:errorcluster)  [unwired: 10 in]
              }
            }
            n156 = Merge Errors(w101, w100) -> (w102:errorcluster)
          }
          event User Event {
            w141 = refnum<class "Abstract.lvclass"> refnum  # Abstract.lvclass
            n157 = event-data() -> ("Timeout"=w135:i32, "Message Data"=w140:variant)  [unwired: 1 in]
            n158 = Variant To Data(error in=w142, type=w141, Variant=w140) -> (data=w137:refnum<class "Abstract.lvclass">, error out=w136:errorcluster)
            n159 = Bundle By Name(cluster=w139, "Abstract.lvclass"=w137) -> (w138:T16)
          }
          event User Event {
            n160 = event-data() -> ("Start Logging?"=w146:bool)  [unwired: 1 in]
            n161 = Bundle By Name(cluster=w149, "Start Logging?"=w146) -> (w147:T16)
          }
          event User Event {
            n162 = event-data() -> ()  [unwired: 1 in, 1 out]
            n163 = Bundle By Name(cluster=T1 {"Message"="", "Data"=[]}, "Message"="Stop") -> (w152:T1)
            n164 = Enqueue Element(queue=w156, element=w152, error in (no error)=w155) -> (queue out=w151:refnum<queue>, error out=w150:errorcluster)  [unwired: 1 in, 1 out]
          }
        }
        n165 = call-dynamic "Delacor_lib_QMH_Error Handler - Message Handling Loop.vi"("error in"=w88, "Message Queue in"=w86) -> ("dup error in"=w87:errorcluster)  [unwired: 8 in, 1 out]
      }
      n166 = while {
        tunnel: w34 -> [w60]
        tunnel: w37 -> [w59]
        tunnel: [w52] -> w35
        tunnel: w33 -> [w51]
        stop <- w54 stop-if-true
        n167 = Dequeue Element(queue=w60, error in (no error)=w59) -> (element=w58:T1, error out=w55:errorcluster)  [unwired: 1 in, 2 out]
        n168 = Unbundle By Name(w58) -> ("Message"=w57:string, "Data"=w56:string[])
        n169 = case shown="Error .." w55 {
          selector: w55 -> [w63 w75]
          tunnel: w57 -> [w65 w76]
          tunnel: w56 -> [w64 _]
          tunnel: [w62 w73] -> w54
          tunnel: [w61 w74] -> w53
          frame No Error {
            n170 = case shown="\"Log Data\", Default" w65 {
              tunnel: w64 -> [_ w71]
              tunnel: w63 -> [w66 w72]
              tunnel: [TRUE FALSE] -> w62
              tunnel: [w66 w69] -> w61
              frame "Stop" {
              }
              frame "Log Data", Default {
                n171 = call "Write Serial Data in tdms.vi"("Command"=Write_Data_Command."Write", "error in (no error)"=w72, "Data"=w71) -> ("error out"=w69:errorcluster)  [unwired: 8 in]
              }
            }
          }
          frame Error {
            n172 = case shown="\"Stop\"" w76 {
              tunnel: w75 -> [w77 w80]
              tunnel: [w77 w80] -> w74
              tunnel: [FALSE TRUE] -> w73
              frame "False", Default {
              }
              frame "Stop" {
              }
            }
          }
        }
        n173 = call-dynamic "Delacor_lib_QMH_Error Handler - Message Handling Loop.vi"("error in"=w53, "Message Queue in"=w51) -> ("dup error in"=w52:errorcluster)  [unwired: 8 in, 1 out]
      }
    }
    frame Error {
      # "Synchronize Caller Events.vi will inform Start Module.vi that the module has launched and will let the code calling Start Module.vi register for broadcasts and would permit the caller receive the broadcast that an error occurred at launch time."
      n174 = call-dynamic "Delacor_lib_QMH_Release Message Queue.vi"("error in"=w454, "Message Queue"=w452) -> ("error out"=w453:errorcluster)  [unwired: 9 in]
      n175 = call "Synchronize Caller Events.vi"("Singleton Module Admin in"=w455) -> ("error out"=w460:errorcluster)  [unwired: 9 in, 1 out]
      n176 = call "Module Name--constant.vi"() -> ("Module Name"=w458:string)  [unwired: 11 in]
      n177 = Format Into String(format string="An error occurred during initialization. %s is no longer running.", w458) -> (resulting string=w456:string)  [unwired: 2 in, 1 out]
      n178 = Merge Errors(w453, w460) -> (w461:errorcluster)
      n179 = call "Error Reported.vi"("Additional Information"=w456, "Error"=w461) -> ()  [unwired: 9 in, 1 out]
    }
  }
  n180 = Merge Errors(w30, w32, w5, w4) -> (w29:errorcluster)
  n181 = call "Close Module.vi"("error in (no error)"=w29, "Module Admin in"=w24) -> ("error out"=w6:errorcluster, "External Launch"=w18:bool, "Module Admin out"=w19:refnum<class "Delacor_lib_QMH_Module Admin.lvclass">)  [unwired: 7 in]
  n182 = Unregister For Events(event registration refnum=w23, error in=w6) -> (error out=w28:errorcluster)
  n183 = Unregister For Events(event registration refnum=w8, error in=w6) -> (error out=w2:errorcluster)
  n184 = Release Queue(queue=w7, error in (no error)=w6) -> (error out=w1:errorcluster)  [unwired: 1 in, 2 out]
  n185 = case "External Launch?" shown="True" w18 {
    tunnel: w28 -> [_ w462]
    frame False {
    }
    frame True {
      n186 = case shown="No Error" w462 {
        frame No Error {
          n187 = invoke class="VI" method="FP.Close"() -> ()  [unwired: 3 in, 3 out]
        }
        frame Error {
          n188 = invoke class="VI" method="FP.Open"("Activate"=TRUE ("Activate?")) -> ()  [unwired: 4 in, 5 out]
        }
      }
    }
  }
  n189 = local write "Module Admin"(w19) -> ()
  n190 = Merge Errors(w28, w2, w1) -> (→"error out":errorcluster)
